vi "Experiment 11.vi"() -> ()   [LabVIEW 2026]
doc: "Experiment 11"
uses:
  <vilib>/Analysis/baseanly.llb/Mean (DBL).vi
  <vilib>/Analysis/NI_AALBase.lvlib
panel:
  out "No. Of Iterations Executed - Loop 10":i32
  out "Output - Loop 10":dbl[](array[numeric]) format="%.3f"
  out "No. Of Iterations Executed - Loop 9":i32
  out "Output - Loop 9":dbl[](array[numeric]) format="%.3f"
  out "No. Of Iterations Executed - Loop 8":i32
  out "Output - Loop 8":dbl[](array[numeric]) format="%.3f"
  out "No. Of Iterations Executed - Loop 7":i32
  out "Output - Loop 7":dbl[](array[numeric]) format="%.3f"
  out "No. Of Iterations Executed - Loop 6":i32
  out "Output - Loop 6":dbl[](array[numeric]) format="%.3f"
  out "No. Of Iterations Executed - Loop 5":i32
  out "Output - Loop 5":dbl[](array[numeric]) format="%.3f"
  out "No. Of Iterations Executed - Loop 4":i32
  out "Output - Loop 4":dbl[](array[numeric]) format="%.3f"
  out "No. Of Iterations Executed - Loop 3":i32
  out "Output - Loop 3":dbl[](array[numeric]) format="%.3f"
  out "Avg. No. Of Iterations Executed - All Loops":dbl format="%.1f"
  out "No. Of Iterations Executed - Loop 2":i32
  out "Output - Loop 2":dbl[](array[numeric]) format="%.3f"
  out "No. Of Iterations Executed - Loop 1":i32
  out "Output - Loop 1":dbl[](array[numeric]) format="%.3f"
  out "Stop VI?":bool
  # "Experiment 11"
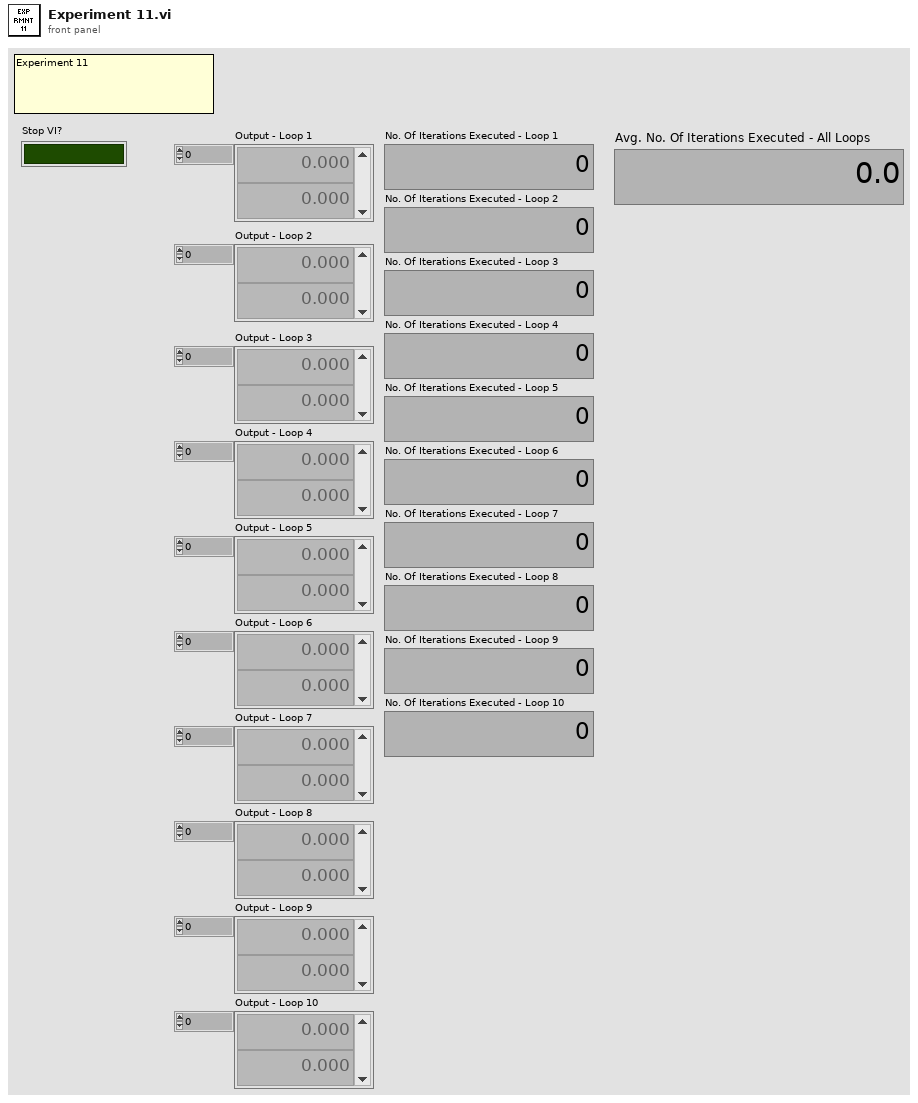
[diagram p1: front panel]
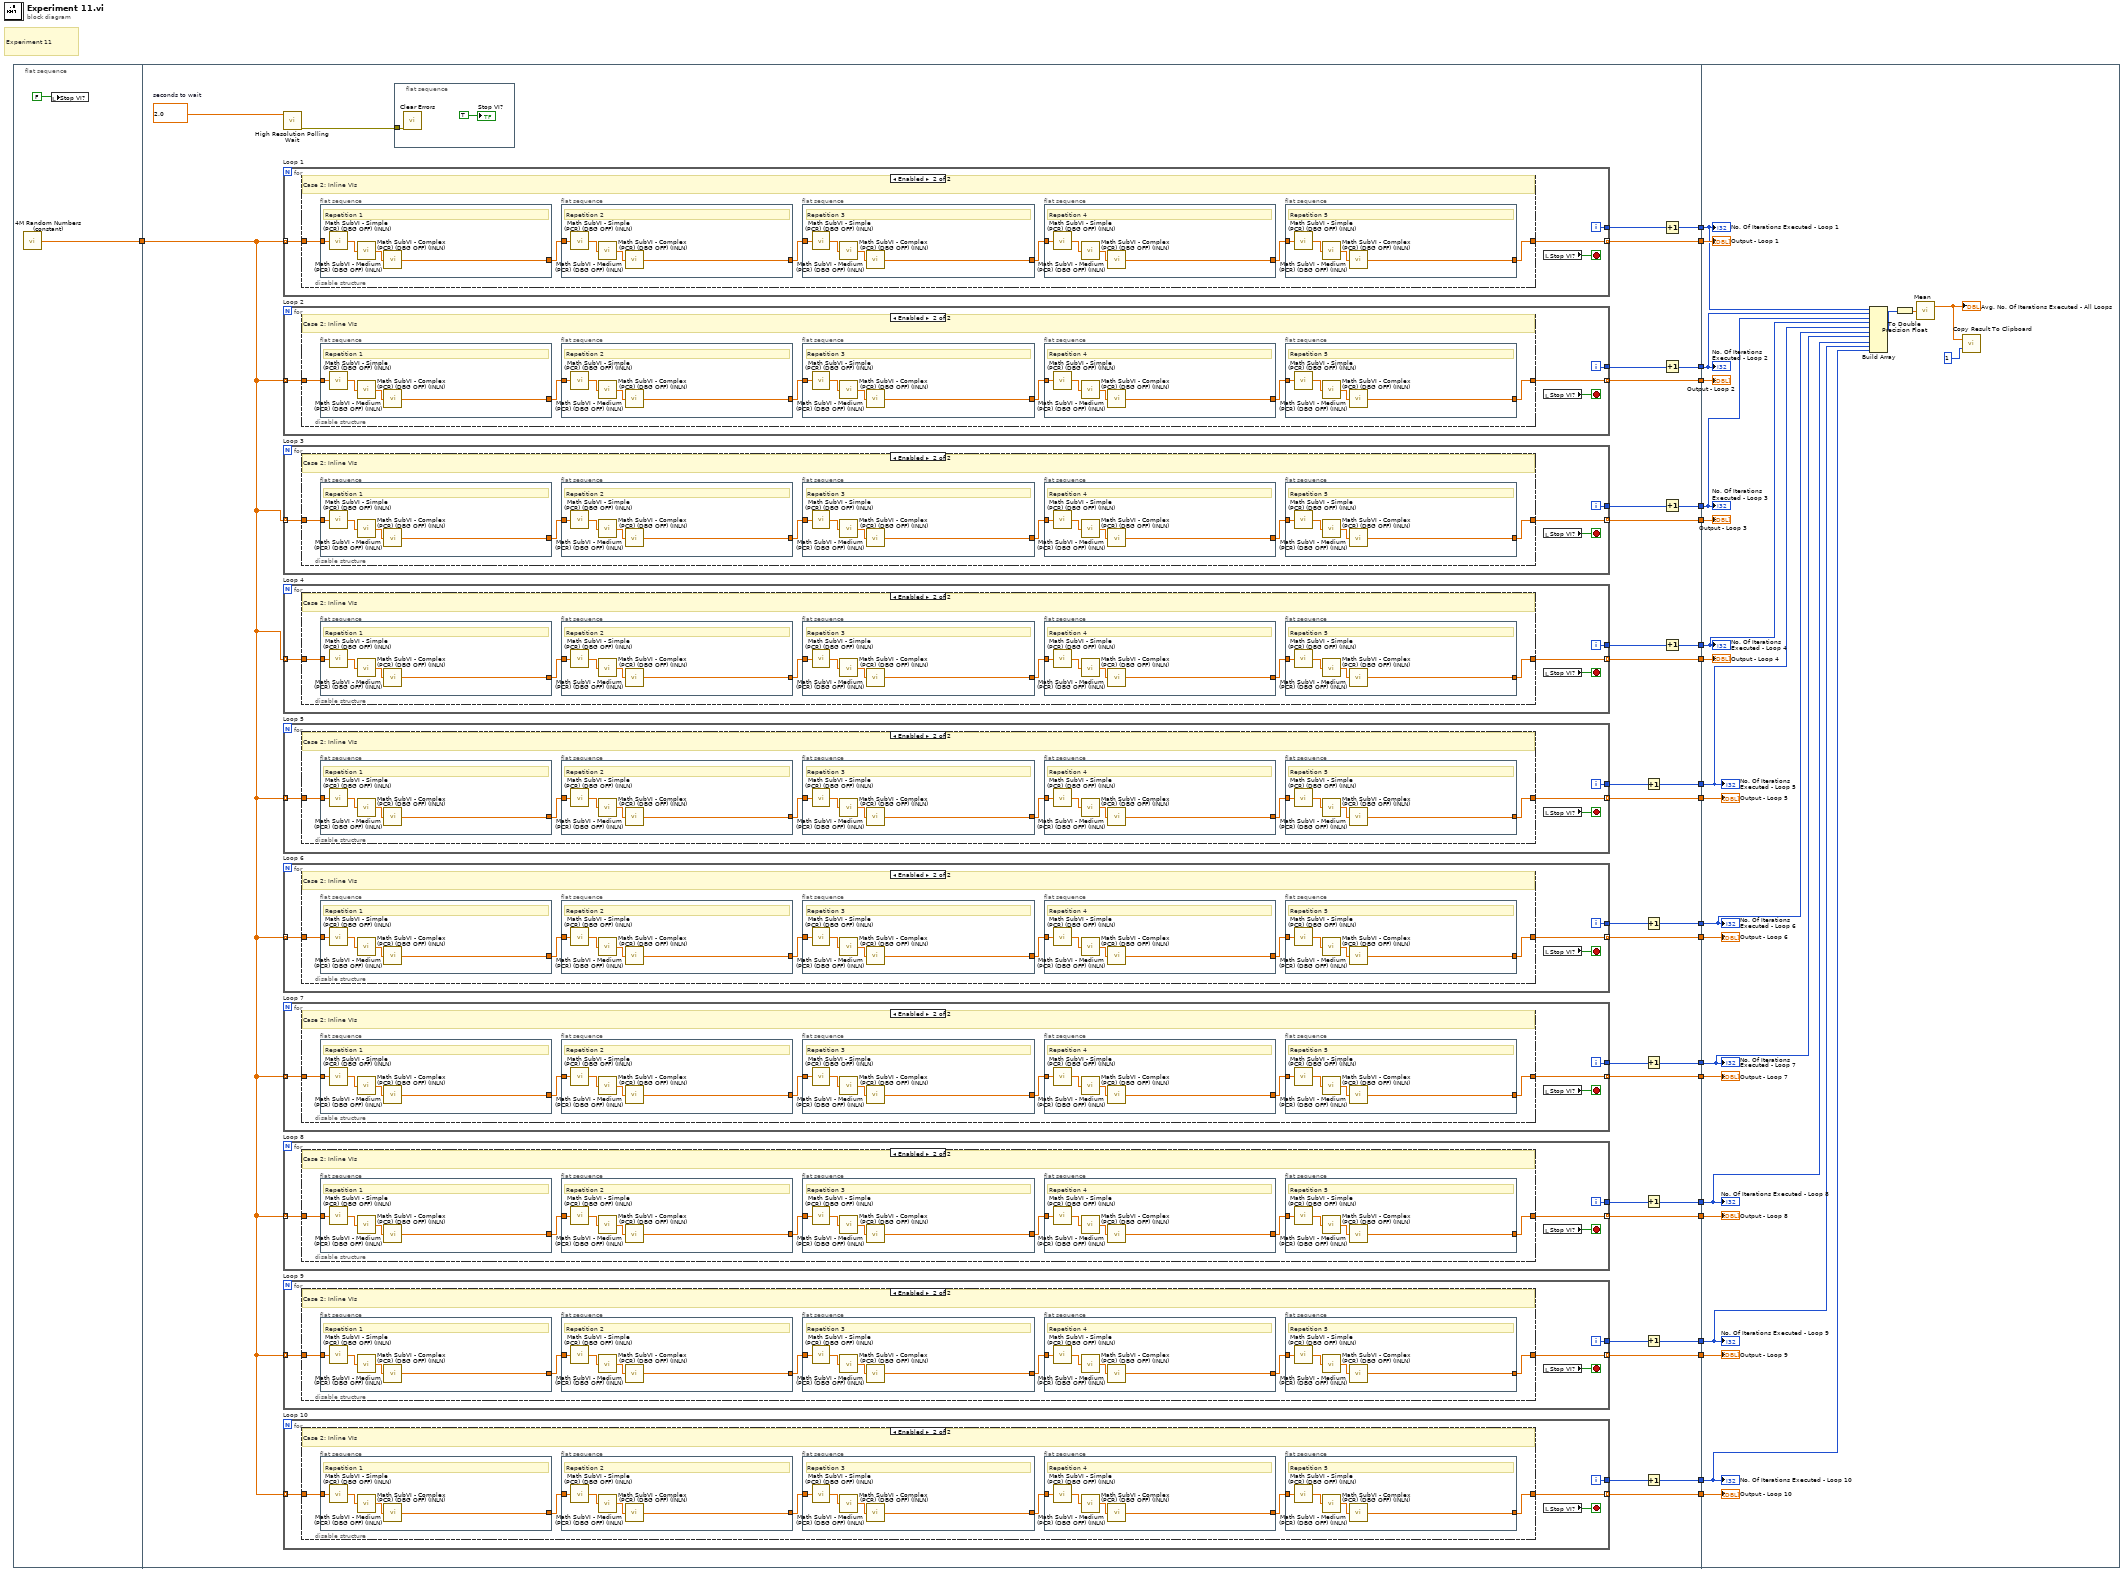
[diagram p0: block diagram]
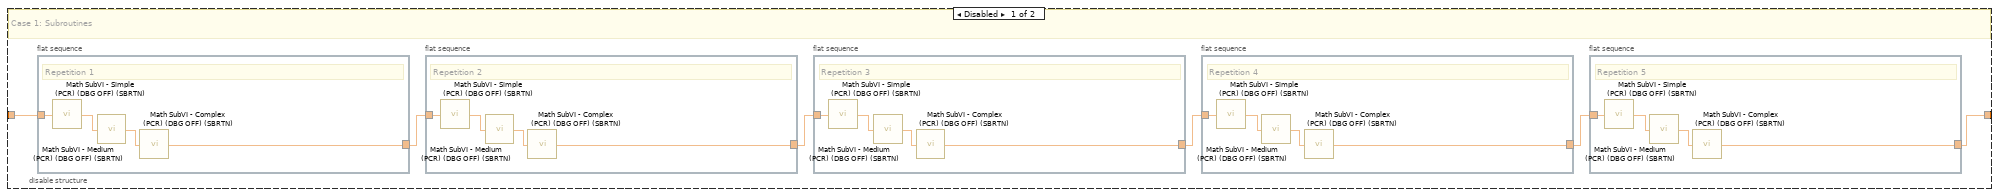
[diagram p2: hidden frame]
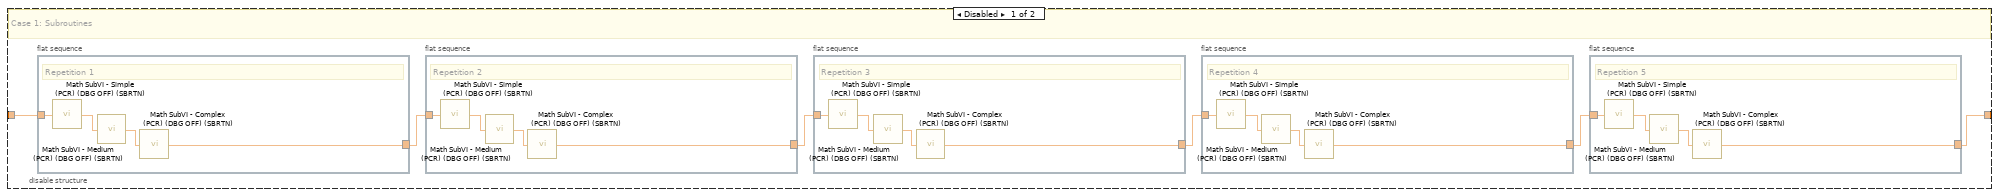
[diagram p3: hidden frame]
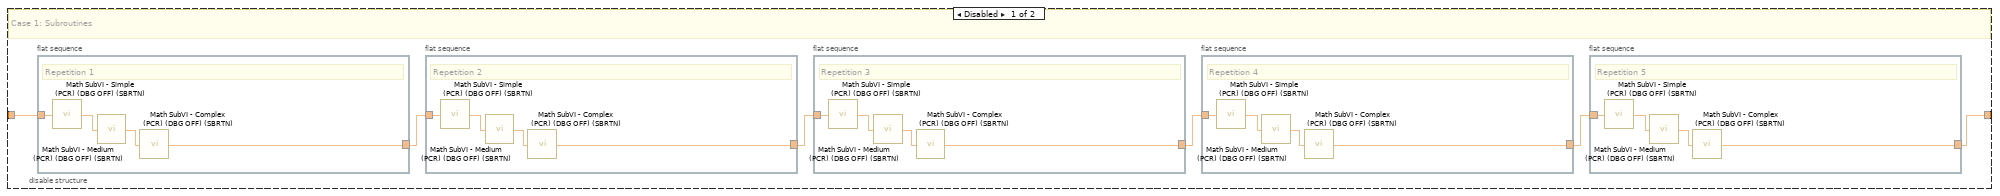
[diagram p4: hidden frame]
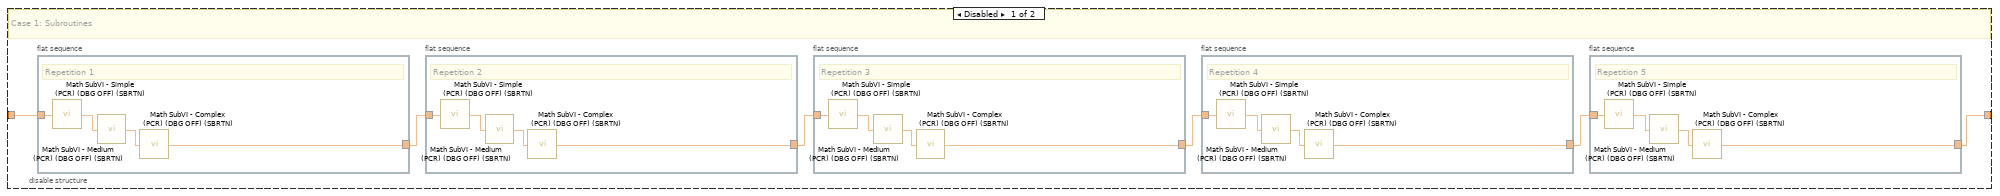
[diagram p5: hidden frame]
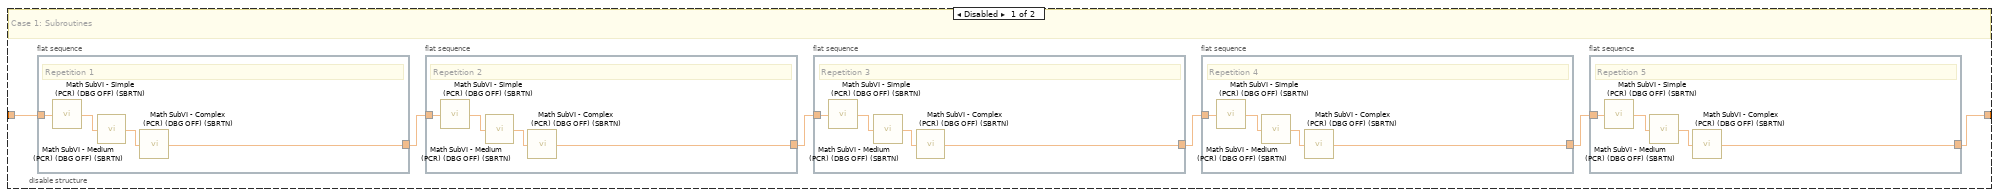
[diagram p6: hidden frame]
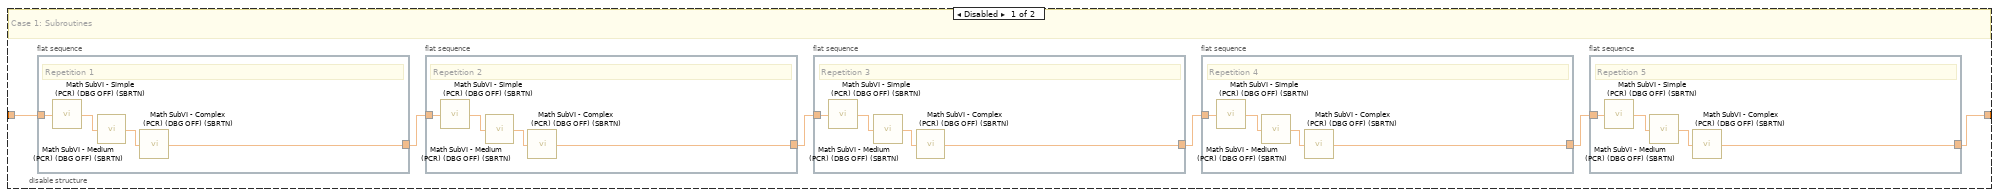
[diagram p7: hidden frame]
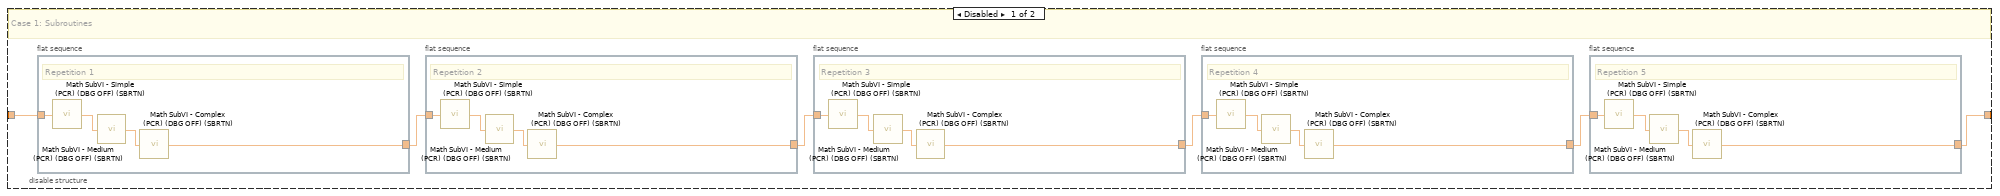
[diagram p8: hidden frame]
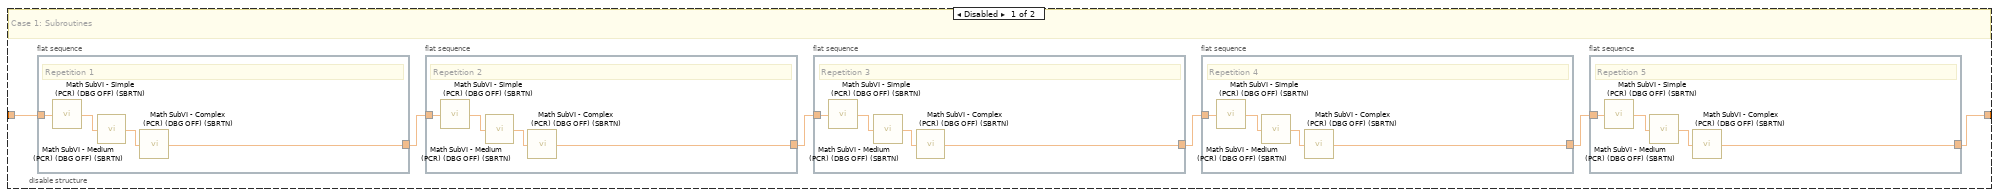
[diagram p9: hidden frame]
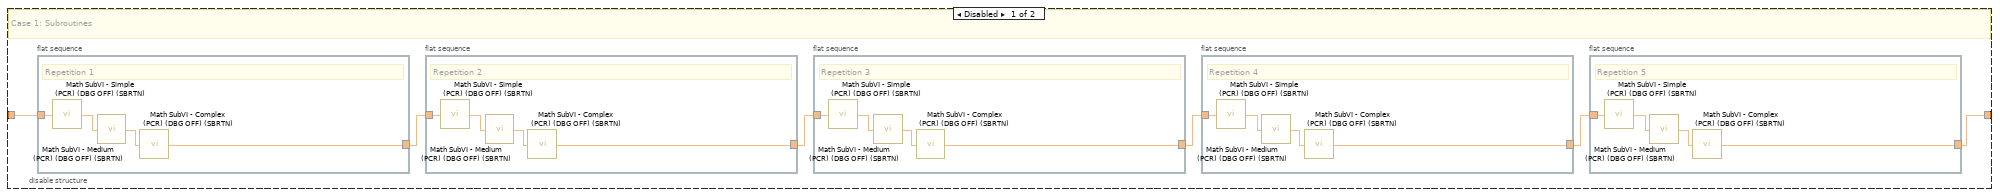
[diagram p10: hidden frame]
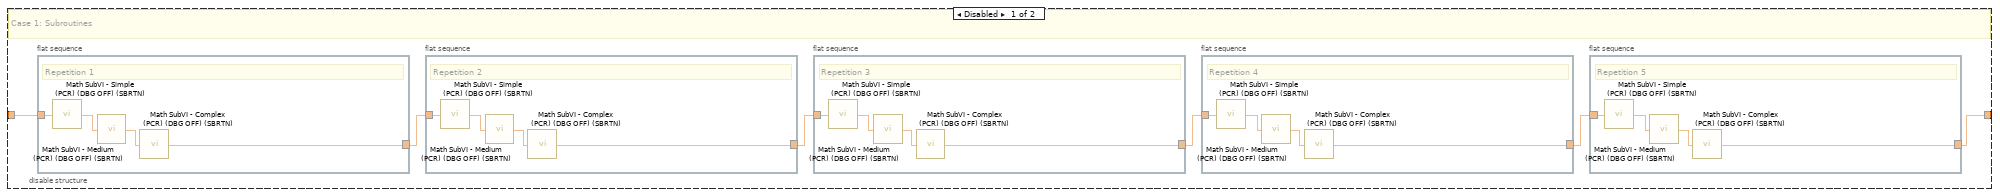
[diagram p11: hidden frame]
diagram:
  # "Experiment 11"
  n1 = flat-sequence {
    tunnel: [w22] -> w13
    tunnel: [w54] -> w21
    tunnel: [w52] -> w20
    tunnel: [w51] -> w19
    tunnel: [w46] -> w18
    tunnel: [w50] -> w17
    tunnel: [w44] -> w16
    tunnel: [w42] -> w15
    tunnel: [w49] -> w14
    tunnel: w13 -> [w48]
    tunnel: [w41] -> w12
    tunnel: [w39] -> w11
    tunnel: [w38] -> w10
    tunnel: [w24] -> w9
    tunnel: [w36] -> w8
    tunnel: [w25] -> w7
    tunnel: [w34] -> w6
    tunnel: [w26] -> w5
    tunnel: [w32] -> w4
    tunnel: [w27] -> w3
    tunnel: [w30] -> w2
    tunnel: [w28] -> w1
    tunnel: w21 -> [w642]
    tunnel: w20 -> [w640]
    tunnel: w19 -> [w639]
    tunnel: w18 -> [w641]
    tunnel: w17 -> [w634]
    tunnel: w16 -> [w637]
    tunnel: w15 -> [w636]
    tunnel: w14 -> [w633]
    tunnel: w12 -> [w630]
    tunnel: w11 -> [w624]
    tunnel: w10 -> [w629]
    tunnel: w9 -> [w623]
    tunnel: w8 -> [w628]
    tunnel: w7 -> [w622]
    tunnel: w6 -> [w627]
    tunnel: w5 -> [w621]
    tunnel: w4 -> [w626]
    tunnel: w3 -> [w620]
    tunnel: w2 -> [w625]
    tunnel: w1 -> [w619]
    frame #0 {
      n2 = call "4M Random Numbers (constant).vi"() -> ("4M Random Numbers"=w22:dbl[])
      n3 = local write "Stop VI?"(FALSE) -> ()
    }
    frame #1 {
      w56 = 2.0  # seconds to wait
      n4 = call <vilib>:"High Resolution Polling Wait.vi"("seconds to wait"=w56) -> ("error out"=w55:errorcluster)  [unwired: 10 in]
      n5 = for "Loop 1" {
        tunnel: w48 -> [w564] mode=indexing
        tunnel: [w561] -> w54 mode=indexing
        tunnel: [w562] -> w53
        i -> [w562]
        stop <- w563 stop-if-true
        n6 = disable-structure shown="Enabled" {
          disable-tunnel: w564 -> [w570 w596]
          disable-tunnel: [w569 w591] -> w561
          frame Disabled {
            # "Case 1: Subroutines"
            n7 = flat-sequence {
              tunnel: w570 -> [w590]
              tunnel: [w587] -> w565
              frame #0 {
                # "Repetition 1"
                n8 = call "Math SubVI - Simple (PCR) (DBG OFF) (SBRTN).vi"("Input"=w590) -> ("Output"=w588:dbl)
                n9 = call "Math SubVI - Medium (PCR) (DBG OFF) (SBRTN).vi"("Input"=w588) -> ("Output"=w589:dbl)
                n10 = call "Math SubVI - Complex (PCR) (DBG OFF) (SBRTN).vi"("Input"=w589) -> ("Output"=w587:dbl)
              }
            }
            n11 = flat-sequence {
              tunnel: w565 -> [w586]
              tunnel: [w583] -> w568
              frame #0 {
                # "Repetition 2"
                n12 = call "Math SubVI - Simple (PCR) (DBG OFF) (SBRTN).vi"("Input"=w586) -> ("Output"=w584:dbl)
                n13 = call "Math SubVI - Medium (PCR) (DBG OFF) (SBRTN).vi"("Input"=w584) -> ("Output"=w585:dbl)
                n14 = call "Math SubVI - Complex (PCR) (DBG OFF) (SBRTN).vi"("Input"=w585) -> ("Output"=w583:dbl)
              }
            }
            n15 = flat-sequence {
              tunnel: w568 -> [w582]
              tunnel: [w579] -> w567
              frame #0 {
                # "Repetition 3"
                n16 = call "Math SubVI - Simple (PCR) (DBG OFF) (SBRTN).vi"("Input"=w582) -> ("Output"=w580:dbl)
                n17 = call "Math SubVI - Medium (PCR) (DBG OFF) (SBRTN).vi"("Input"=w580) -> ("Output"=w581:dbl)
                n18 = call "Math SubVI - Complex (PCR) (DBG OFF) (SBRTN).vi"("Input"=w581) -> ("Output"=w579:dbl)
              }
            }
            n19 = flat-sequence {
              tunnel: w567 -> [w578]
              tunnel: [w575] -> w566
              frame #0 {
                # "Repetition 4"
                n20 = call "Math SubVI - Simple (PCR) (DBG OFF) (SBRTN).vi"("Input"=w578) -> ("Output"=w576:dbl)
                n21 = call "Math SubVI - Medium (PCR) (DBG OFF) (SBRTN).vi"("Input"=w576) -> ("Output"=w577:dbl)
                n22 = call "Math SubVI - Complex (PCR) (DBG OFF) (SBRTN).vi"("Input"=w577) -> ("Output"=w575:dbl)
              }
            }
            n23 = flat-sequence {
              tunnel: w566 -> [w574]
              tunnel: [w571] -> w569
              frame #0 {
                # "Repetition 5"
                n24 = call "Math SubVI - Simple (PCR) (DBG OFF) (SBRTN).vi"("Input"=w574) -> ("Output"=w572:dbl)
                n25 = call "Math SubVI - Medium (PCR) (DBG OFF) (SBRTN).vi"("Input"=w572) -> ("Output"=w573:dbl)
                n26 = call "Math SubVI - Complex (PCR) (DBG OFF) (SBRTN).vi"("Input"=w573) -> ("Output"=w571:dbl)
              }
            }
          }
          frame Enabled {
            # "Case 2: Inline VIs"
            n27 = flat-sequence {
              tunnel: w596 -> [w616]
              tunnel: [w613] -> w595
              frame #0 {
                # "Repetition 1"
                n28 = call "Math SubVI - Simple (PCR) (DBG OFF) (INLN).vi"("Input"=w616) -> ("Output"=w614:dbl)
                n29 = call "Math SubVI - Medium (PCR) (DBG OFF) (INLN).vi"("Input"=w614) -> ("Output"=w615:dbl)
                n30 = call "Math SubVI - Complex (PCR) (DBG OFF) (INLN).vi"("Input"=w615) -> ("Output"=w613:dbl)
              }
            }
            n31 = flat-sequence {
              tunnel: w595 -> [w612]
              tunnel: [w609] -> w594
              frame #0 {
                # "Repetition 2"
                n32 = call "Math SubVI - Simple (PCR) (DBG OFF) (INLN).vi"("Input"=w612) -> ("Output"=w610:dbl)
                n33 = call "Math SubVI - Medium (PCR) (DBG OFF) (INLN).vi"("Input"=w610) -> ("Output"=w611:dbl)
                n34 = call "Math SubVI - Complex (PCR) (DBG OFF) (INLN).vi"("Input"=w611) -> ("Output"=w609:dbl)
              }
            }
            n35 = flat-sequence {
              tunnel: w594 -> [w608]
              tunnel: [w605] -> w593
              frame #0 {
                # "Repetition 3"
                n36 = call "Math SubVI - Simple (PCR) (DBG OFF) (INLN).vi"("Input"=w608) -> ("Output"=w606:dbl)
                n37 = call "Math SubVI - Medium (PCR) (DBG OFF) (INLN).vi"("Input"=w606) -> ("Output"=w607:dbl)
                n38 = call "Math SubVI - Complex (PCR) (DBG OFF) (INLN).vi"("Input"=w607) -> ("Output"=w605:dbl)
              }
            }
            n39 = flat-sequence {
              tunnel: w593 -> [w604]
              tunnel: [w601] -> w592
              frame #0 {
                # "Repetition 4"
                n40 = call "Math SubVI - Simple (PCR) (DBG OFF) (INLN).vi"("Input"=w604) -> ("Output"=w602:dbl)
                n41 = call "Math SubVI - Medium (PCR) (DBG OFF) (INLN).vi"("Input"=w602) -> ("Output"=w603:dbl)
                n42 = call "Math SubVI - Complex (PCR) (DBG OFF) (INLN).vi"("Input"=w603) -> ("Output"=w601:dbl)
              }
            }
            n43 = flat-sequence {
              tunnel: w592 -> [w600]
              tunnel: [w597] -> w591
              frame #0 {
                # "Repetition 5"
                n44 = call "Math SubVI - Simple (PCR) (DBG OFF) (INLN).vi"("Input"=w600) -> ("Output"=w598:dbl)
                n45 = call "Math SubVI - Medium (PCR) (DBG OFF) (INLN).vi"("Input"=w598) -> ("Output"=w599:dbl)
                n46 = call "Math SubVI - Complex (PCR) (DBG OFF) (INLN).vi"("Input"=w599) -> ("Output"=w597:dbl)
              }
            }
          }
        }
        n47 = local read "Stop VI?"() -> (w563:bool)
      }
      n48 = for "Loop 2" {
        tunnel: w48 -> [w508] mode=indexing
        tunnel: [w505] -> w46 mode=indexing
        tunnel: [w506] -> w47
        i -> [w506]
        stop <- w507 stop-if-true
        n49 = disable-structure shown="Enabled" {
          disable-tunnel: w508 -> [w514 w540]
          disable-tunnel: [w513 w535] -> w505
          frame Disabled {
            # "Case 1: Subroutines"
            n50 = flat-sequence {
              tunnel: w514 -> [w534]
              tunnel: [w531] -> w509
              frame #0 {
                # "Repetition 1"
                n51 = call "Math SubVI - Simple (PCR) (DBG OFF) (SBRTN).vi"("Input"=w534) -> ("Output"=w532:dbl)
                n52 = call "Math SubVI - Medium (PCR) (DBG OFF) (SBRTN).vi"("Input"=w532) -> ("Output"=w533:dbl)
                n53 = call "Math SubVI - Complex (PCR) (DBG OFF) (SBRTN).vi"("Input"=w533) -> ("Output"=w531:dbl)
              }
            }
            n54 = flat-sequence {
              tunnel: w509 -> [w530]
              tunnel: [w527] -> w512
              frame #0 {
                # "Repetition 2"
                n55 = call "Math SubVI - Simple (PCR) (DBG OFF) (SBRTN).vi"("Input"=w530) -> ("Output"=w528:dbl)
                n56 = call "Math SubVI - Medium (PCR) (DBG OFF) (SBRTN).vi"("Input"=w528) -> ("Output"=w529:dbl)
                n57 = call "Math SubVI - Complex (PCR) (DBG OFF) (SBRTN).vi"("Input"=w529) -> ("Output"=w527:dbl)
              }
            }
            n58 = flat-sequence {
              tunnel: w512 -> [w526]
              tunnel: [w523] -> w511
              frame #0 {
                # "Repetition 3"
                n59 = call "Math SubVI - Simple (PCR) (DBG OFF) (SBRTN).vi"("Input"=w526) -> ("Output"=w524:dbl)
                n60 = call "Math SubVI - Medium (PCR) (DBG OFF) (SBRTN).vi"("Input"=w524) -> ("Output"=w525:dbl)
                n61 = call "Math SubVI - Complex (PCR) (DBG OFF) (SBRTN).vi"("Input"=w525) -> ("Output"=w523:dbl)
              }
            }
            n62 = flat-sequence {
              tunnel: w511 -> [w522]
              tunnel: [w519] -> w510
              frame #0 {
                # "Repetition 4"
                n63 = call "Math SubVI - Simple (PCR) (DBG OFF) (SBRTN).vi"("Input"=w522) -> ("Output"=w520:dbl)
                n64 = call "Math SubVI - Medium (PCR) (DBG OFF) (SBRTN).vi"("Input"=w520) -> ("Output"=w521:dbl)
                n65 = call "Math SubVI - Complex (PCR) (DBG OFF) (SBRTN).vi"("Input"=w521) -> ("Output"=w519:dbl)
              }
            }
            n66 = flat-sequence {
              tunnel: w510 -> [w518]
              tunnel: [w515] -> w513
              frame #0 {
                # "Repetition 5"
                n67 = call "Math SubVI - Simple (PCR) (DBG OFF) (SBRTN).vi"("Input"=w518) -> ("Output"=w516:dbl)
                n68 = call "Math SubVI - Medium (PCR) (DBG OFF) (SBRTN).vi"("Input"=w516) -> ("Output"=w517:dbl)
                n69 = call "Math SubVI - Complex (PCR) (DBG OFF) (SBRTN).vi"("Input"=w517) -> ("Output"=w515:dbl)
              }
            }
          }
          frame Enabled {
            # "Case 2: Inline VIs"
            n70 = flat-sequence {
              tunnel: w540 -> [w560]
              tunnel: [w557] -> w539
              frame #0 {
                # "Repetition 1"
                n71 = call "Math SubVI - Simple (PCR) (DBG OFF) (INLN).vi"("Input"=w560) -> ("Output"=w558:dbl)
                n72 = call "Math SubVI - Medium (PCR) (DBG OFF) (INLN).vi"("Input"=w558) -> ("Output"=w559:dbl)
                n73 = call "Math SubVI - Complex (PCR) (DBG OFF) (INLN).vi"("Input"=w559) -> ("Output"=w557:dbl)
              }
            }
            n74 = flat-sequence {
              tunnel: w539 -> [w556]
              tunnel: [w553] -> w538
              frame #0 {
                # "Repetition 2"
                n75 = call "Math SubVI - Simple (PCR) (DBG OFF) (INLN).vi"("Input"=w556) -> ("Output"=w554:dbl)
                n76 = call "Math SubVI - Medium (PCR) (DBG OFF) (INLN).vi"("Input"=w554) -> ("Output"=w555:dbl)
                n77 = call "Math SubVI - Complex (PCR) (DBG OFF) (INLN).vi"("Input"=w555) -> ("Output"=w553:dbl)
              }
            }
            n78 = flat-sequence {
              tunnel: w538 -> [w552]
              tunnel: [w549] -> w537
              frame #0 {
                # "Repetition 3"
                n79 = call "Math SubVI - Simple (PCR) (DBG OFF) (INLN).vi"("Input"=w552) -> ("Output"=w550:dbl)
                n80 = call "Math SubVI - Medium (PCR) (DBG OFF) (INLN).vi"("Input"=w550) -> ("Output"=w551:dbl)
                n81 = call "Math SubVI - Complex (PCR) (DBG OFF) (INLN).vi"("Input"=w551) -> ("Output"=w549:dbl)
              }
            }
            n82 = flat-sequence {
              tunnel: w537 -> [w548]
              tunnel: [w545] -> w536
              frame #0 {
                # "Repetition 4"
                n83 = call "Math SubVI - Simple (PCR) (DBG OFF) (INLN).vi"("Input"=w548) -> ("Output"=w546:dbl)
                n84 = call "Math SubVI - Medium (PCR) (DBG OFF) (INLN).vi"("Input"=w546) -> ("Output"=w547:dbl)
                n85 = call "Math SubVI - Complex (PCR) (DBG OFF) (INLN).vi"("Input"=w547) -> ("Output"=w545:dbl)
              }
            }
            n86 = flat-sequence {
              tunnel: w536 -> [w544]
              tunnel: [w541] -> w535
              frame #0 {
                # "Repetition 5"
                n87 = call "Math SubVI - Simple (PCR) (DBG OFF) (INLN).vi"("Input"=w544) -> ("Output"=w542:dbl)
                n88 = call "Math SubVI - Medium (PCR) (DBG OFF) (INLN).vi"("Input"=w542) -> ("Output"=w543:dbl)
                n89 = call "Math SubVI - Complex (PCR) (DBG OFF) (INLN).vi"("Input"=w543) -> ("Output"=w541:dbl)
              }
            }
          }
        }
        n90 = local read "Stop VI?"() -> (w507:bool)
      }
      n91 = for "Loop 3" {
        tunnel: w48 -> [w452] mode=indexing
        tunnel: [w449] -> w44 mode=indexing
        tunnel: [w450] -> w45
        i -> [w450]
        stop <- w451 stop-if-true
        n92 = disable-structure shown="Enabled" {
          disable-tunnel: w452 -> [w458 w484]
          disable-tunnel: [w457 w479] -> w449
          frame Disabled {
            # "Case 1: Subroutines"
            n93 = flat-sequence {
              tunnel: w458 -> [w478]
              tunnel: [w475] -> w453
              frame #0 {
                # "Repetition 1"
                n94 = call "Math SubVI - Simple (PCR) (DBG OFF) (SBRTN).vi"("Input"=w478) -> ("Output"=w476:dbl)
                n95 = call "Math SubVI - Medium (PCR) (DBG OFF) (SBRTN).vi"("Input"=w476) -> ("Output"=w477:dbl)
                n96 = call "Math SubVI - Complex (PCR) (DBG OFF) (SBRTN).vi"("Input"=w477) -> ("Output"=w475:dbl)
              }
            }
            n97 = flat-sequence {
              tunnel: w453 -> [w474]
              tunnel: [w471] -> w456
              frame #0 {
                # "Repetition 2"
                n98 = call "Math SubVI - Simple (PCR) (DBG OFF) (SBRTN).vi"("Input"=w474) -> ("Output"=w472:dbl)
                n99 = call "Math SubVI - Medium (PCR) (DBG OFF) (SBRTN).vi"("Input"=w472) -> ("Output"=w473:dbl)
                n100 = call "Math SubVI - Complex (PCR) (DBG OFF) (SBRTN).vi"("Input"=w473) -> ("Output"=w471:dbl)
              }
            }
            n101 = flat-sequence {
              tunnel: w456 -> [w470]
              tunnel: [w467] -> w455
              frame #0 {
                # "Repetition 3"
                n102 = call "Math SubVI - Simple (PCR) (DBG OFF) (SBRTN).vi"("Input"=w470) -> ("Output"=w468:dbl)
                n103 = call "Math SubVI - Medium (PCR) (DBG OFF) (SBRTN).vi"("Input"=w468) -> ("Output"=w469:dbl)
                n104 = call "Math SubVI - Complex (PCR) (DBG OFF) (SBRTN).vi"("Input"=w469) -> ("Output"=w467:dbl)
              }
            }
            n105 = flat-sequence {
              tunnel: w455 -> [w466]
              tunnel: [w463] -> w454
              frame #0 {
                # "Repetition 4"
                n106 = call "Math SubVI - Simple (PCR) (DBG OFF) (SBRTN).vi"("Input"=w466) -> ("Output"=w464:dbl)
                n107 = call "Math SubVI - Medium (PCR) (DBG OFF) (SBRTN).vi"("Input"=w464) -> ("Output"=w465:dbl)
                n108 = call "Math SubVI - Complex (PCR) (DBG OFF) (SBRTN).vi"("Input"=w465) -> ("Output"=w463:dbl)
              }
            }
            n109 = flat-sequence {
              tunnel: w454 -> [w462]
              tunnel: [w459] -> w457
              frame #0 {
                # "Repetition 5"
                n110 = call "Math SubVI - Simple (PCR) (DBG OFF) (SBRTN).vi"("Input"=w462) -> ("Output"=w460:dbl)
                n111 = call "Math SubVI - Medium (PCR) (DBG OFF) (SBRTN).vi"("Input"=w460) -> ("Output"=w461:dbl)
                n112 = call "Math SubVI - Complex (PCR) (DBG OFF) (SBRTN).vi"("Input"=w461) -> ("Output"=w459:dbl)
              }
            }
          }
          frame Enabled {
            # "Case 2: Inline VIs"
            n113 = flat-sequence {
              tunnel: w484 -> [w504]
              tunnel: [w501] -> w483
              frame #0 {
                # "Repetition 1"
                n114 = call "Math SubVI - Simple (PCR) (DBG OFF) (INLN).vi"("Input"=w504) -> ("Output"=w502:dbl)
                n115 = call "Math SubVI - Medium (PCR) (DBG OFF) (INLN).vi"("Input"=w502) -> ("Output"=w503:dbl)
                n116 = call "Math SubVI - Complex (PCR) (DBG OFF) (INLN).vi"("Input"=w503) -> ("Output"=w501:dbl)
              }
            }
            n117 = flat-sequence {
              tunnel: w483 -> [w500]
              tunnel: [w497] -> w482
              frame #0 {
                # "Repetition 2"
                n118 = call "Math SubVI - Simple (PCR) (DBG OFF) (INLN).vi"("Input"=w500) -> ("Output"=w498:dbl)
                n119 = call "Math SubVI - Medium (PCR) (DBG OFF) (INLN).vi"("Input"=w498) -> ("Output"=w499:dbl)
                n120 = call "Math SubVI - Complex (PCR) (DBG OFF) (INLN).vi"("Input"=w499) -> ("Output"=w497:dbl)
              }
            }
            n121 = flat-sequence {
              tunnel: w482 -> [w496]
              tunnel: [w493] -> w481
              frame #0 {
                # "Repetition 3"
                n122 = call "Math SubVI - Simple (PCR) (DBG OFF) (INLN).vi"("Input"=w496) -> ("Output"=w494:dbl)
                n123 = call "Math SubVI - Medium (PCR) (DBG OFF) (INLN).vi"("Input"=w494) -> ("Output"=w495:dbl)
                n124 = call "Math SubVI - Complex (PCR) (DBG OFF) (INLN).vi"("Input"=w495) -> ("Output"=w493:dbl)
              }
            }
            n125 = flat-sequence {
              tunnel: w481 -> [w492]
              tunnel: [w489] -> w480
              frame #0 {
                # "Repetition 4"
                n126 = call "Math SubVI - Simple (PCR) (DBG OFF) (INLN).vi"("Input"=w492) -> ("Output"=w490:dbl)
                n127 = call "Math SubVI - Medium (PCR) (DBG OFF) (INLN).vi"("Input"=w490) -> ("Output"=w491:dbl)
                n128 = call "Math SubVI - Complex (PCR) (DBG OFF) (INLN).vi"("Input"=w491) -> ("Output"=w489:dbl)
              }
            }
            n129 = flat-sequence {
              tunnel: w480 -> [w488]
              tunnel: [w485] -> w479
              frame #0 {
                # "Repetition 5"
                n130 = call "Math SubVI - Simple (PCR) (DBG OFF) (INLN).vi"("Input"=w488) -> ("Output"=w486:dbl)
                n131 = call "Math SubVI - Medium (PCR) (DBG OFF) (INLN).vi"("Input"=w486) -> ("Output"=w487:dbl)
                n132 = call "Math SubVI - Complex (PCR) (DBG OFF) (INLN).vi"("Input"=w487) -> ("Output"=w485:dbl)
              }
            }
          }
        }
        n133 = local read "Stop VI?"() -> (w451:bool)
      }
      n134 = for "Loop 4" {
        tunnel: w48 -> [w396] mode=indexing
        tunnel: [w393] -> w42 mode=indexing
        tunnel: [w394] -> w43
        i -> [w394]
        stop <- w395 stop-if-true
        n135 = disable-structure shown="Enabled" {
          disable-tunnel: w396 -> [w402 w428]
          disable-tunnel: [w401 w423] -> w393
          frame Disabled {
            # "Case 1: Subroutines"
            n136 = flat-sequence {
              tunnel: w402 -> [w422]
              tunnel: [w419] -> w397
              frame #0 {
                # "Repetition 1"
                n137 = call "Math SubVI - Simple (PCR) (DBG OFF) (SBRTN).vi"("Input"=w422) -> ("Output"=w420:dbl)
                n138 = call "Math SubVI - Medium (PCR) (DBG OFF) (SBRTN).vi"("Input"=w420) -> ("Output"=w421:dbl)
                n139 = call "Math SubVI - Complex (PCR) (DBG OFF) (SBRTN).vi"("Input"=w421) -> ("Output"=w419:dbl)
              }
            }
            n140 = flat-sequence {
              tunnel: w397 -> [w418]
              tunnel: [w415] -> w400
              frame #0 {
                # "Repetition 2"
                n141 = call "Math SubVI - Simple (PCR) (DBG OFF) (SBRTN).vi"("Input"=w418) -> ("Output"=w416:dbl)
                n142 = call "Math SubVI - Medium (PCR) (DBG OFF) (SBRTN).vi"("Input"=w416) -> ("Output"=w417:dbl)
                n143 = call "Math SubVI - Complex (PCR) (DBG OFF) (SBRTN).vi"("Input"=w417) -> ("Output"=w415:dbl)
              }
            }
            n144 = flat-sequence {
              tunnel: w400 -> [w414]
              tunnel: [w411] -> w399
              frame #0 {
                # "Repetition 3"
                n145 = call "Math SubVI - Simple (PCR) (DBG OFF) (SBRTN).vi"("Input"=w414) -> ("Output"=w412:dbl)
                n146 = call "Math SubVI - Medium (PCR) (DBG OFF) (SBRTN).vi"("Input"=w412) -> ("Output"=w413:dbl)
                n147 = call "Math SubVI - Complex (PCR) (DBG OFF) (SBRTN).vi"("Input"=w413) -> ("Output"=w411:dbl)
              }
            }
            n148 = flat-sequence {
              tunnel: w399 -> [w410]
              tunnel: [w407] -> w398
              frame #0 {
                # "Repetition 4"
                n149 = call "Math SubVI - Simple (PCR) (DBG OFF) (SBRTN).vi"("Input"=w410) -> ("Output"=w408:dbl)
                n150 = call "Math SubVI - Medium (PCR) (DBG OFF) (SBRTN).vi"("Input"=w408) -> ("Output"=w409:dbl)
                n151 = call "Math SubVI - Complex (PCR) (DBG OFF) (SBRTN).vi"("Input"=w409) -> ("Output"=w407:dbl)
              }
            }
            n152 = flat-sequence {
              tunnel: w398 -> [w406]
              tunnel: [w403] -> w401
              frame #0 {
                # "Repetition 5"
                n153 = call "Math SubVI - Simple (PCR) (DBG OFF) (SBRTN).vi"("Input"=w406) -> ("Output"=w404:dbl)
                n154 = call "Math SubVI - Medium (PCR) (DBG OFF) (SBRTN).vi"("Input"=w404) -> ("Output"=w405:dbl)
                n155 = call "Math SubVI - Complex (PCR) (DBG OFF) (SBRTN).vi"("Input"=w405) -> ("Output"=w403:dbl)
              }
            }
          }
          frame Enabled {
            # "Case 2: Inline VIs"
            n156 = flat-sequence {
              tunnel: w428 -> [w448]
              tunnel: [w445] -> w427
              frame #0 {
                # "Repetition 1"
                n157 = call "Math SubVI - Simple (PCR) (DBG OFF) (INLN).vi"("Input"=w448) -> ("Output"=w446:dbl)
                n158 = call "Math SubVI - Medium (PCR) (DBG OFF) (INLN).vi"("Input"=w446) -> ("Output"=w447:dbl)
                n159 = call "Math SubVI - Complex (PCR) (DBG OFF) (INLN).vi"("Input"=w447) -> ("Output"=w445:dbl)
              }
            }
            n160 = flat-sequence {
              tunnel: w427 -> [w444]
              tunnel: [w441] -> w426
              frame #0 {
                # "Repetition 2"
                n161 = call "Math SubVI - Simple (PCR) (DBG OFF) (INLN).vi"("Input"=w444) -> ("Output"=w442:dbl)
                n162 = call "Math SubVI - Medium (PCR) (DBG OFF) (INLN).vi"("Input"=w442) -> ("Output"=w443:dbl)
                n163 = call "Math SubVI - Complex (PCR) (DBG OFF) (INLN).vi"("Input"=w443) -> ("Output"=w441:dbl)
              }
            }
            n164 = flat-sequence {
              tunnel: w426 -> [w440]
              tunnel: [w437] -> w425
              frame #0 {
                # "Repetition 3"
                n165 = call "Math SubVI - Simple (PCR) (DBG OFF) (INLN).vi"("Input"=w440) -> ("Output"=w438:dbl)
                n166 = call "Math SubVI - Medium (PCR) (DBG OFF) (INLN).vi"("Input"=w438) -> ("Output"=w439:dbl)
                n167 = call "Math SubVI - Complex (PCR) (DBG OFF) (INLN).vi"("Input"=w439) -> ("Output"=w437:dbl)
              }
            }
            n168 = flat-sequence {
              tunnel: w425 -> [w436]
              tunnel: [w433] -> w424
              frame #0 {
                # "Repetition 4"
                n169 = call "Math SubVI - Simple (PCR) (DBG OFF) (INLN).vi"("Input"=w436) -> ("Output"=w434:dbl)
                n170 = call "Math SubVI - Medium (PCR) (DBG OFF) (INLN).vi"("Input"=w434) -> ("Output"=w435:dbl)
                n171 = call "Math SubVI - Complex (PCR) (DBG OFF) (INLN).vi"("Input"=w435) -> ("Output"=w433:dbl)
              }
            }
            n172 = flat-sequence {
              tunnel: w424 -> [w432]
              tunnel: [w429] -> w423
              frame #0 {
                # "Repetition 5"
                n173 = call "Math SubVI - Simple (PCR) (DBG OFF) (INLN).vi"("Input"=w432) -> ("Output"=w430:dbl)
                n174 = call "Math SubVI - Medium (PCR) (DBG OFF) (INLN).vi"("Input"=w430) -> ("Output"=w431:dbl)
                n175 = call "Math SubVI - Complex (PCR) (DBG OFF) (INLN).vi"("Input"=w431) -> ("Output"=w429:dbl)
              }
            }
          }
        }
        n176 = local read "Stop VI?"() -> (w395:bool)
      }
      n177 = for "Loop 5" {
        tunnel: w48 -> [w340] mode=indexing
        tunnel: [w337] -> w41 mode=indexing
        tunnel: [w338] -> w40
        i -> [w338]
        stop <- w339 stop-if-true
        n178 = disable-structure shown="Enabled" {
          disable-tunnel: w340 -> [w346 w372]
          disable-tunnel: [w345 w367] -> w337
          frame Disabled {
            # "Case 1: Subroutines"
            n179 = flat-sequence {
              tunnel: w346 -> [w366]
              tunnel: [w363] -> w341
              frame #0 {
                # "Repetition 1"
                n180 = call "Math SubVI - Simple (PCR) (DBG OFF) (SBRTN).vi"("Input"=w366) -> ("Output"=w364:dbl)
                n181 = call "Math SubVI - Medium (PCR) (DBG OFF) (SBRTN).vi"("Input"=w364) -> ("Output"=w365:dbl)
                n182 = call "Math SubVI - Complex (PCR) (DBG OFF) (SBRTN).vi"("Input"=w365) -> ("Output"=w363:dbl)
              }
            }
            n183 = flat-sequence {
              tunnel: w341 -> [w362]
              tunnel: [w359] -> w344
              frame #0 {
                # "Repetition 2"
                n184 = call "Math SubVI - Simple (PCR) (DBG OFF) (SBRTN).vi"("Input"=w362) -> ("Output"=w360:dbl)
                n185 = call "Math SubVI - Medium (PCR) (DBG OFF) (SBRTN).vi"("Input"=w360) -> ("Output"=w361:dbl)
                n186 = call "Math SubVI - Complex (PCR) (DBG OFF) (SBRTN).vi"("Input"=w361) -> ("Output"=w359:dbl)
              }
            }
            n187 = flat-sequence {
              tunnel: w344 -> [w358]
              tunnel: [w355] -> w343
              frame #0 {
                # "Repetition 3"
                n188 = call "Math SubVI - Simple (PCR) (DBG OFF) (SBRTN).vi"("Input"=w358) -> ("Output"=w356:dbl)
                n189 = call "Math SubVI - Medium (PCR) (DBG OFF) (SBRTN).vi"("Input"=w356) -> ("Output"=w357:dbl)
                n190 = call "Math SubVI - Complex (PCR) (DBG OFF) (SBRTN).vi"("Input"=w357) -> ("Output"=w355:dbl)
              }
            }
            n191 = flat-sequence {
              tunnel: w343 -> [w354]
              tunnel: [w351] -> w342
              frame #0 {
                # "Repetition 4"
                n192 = call "Math SubVI - Simple (PCR) (DBG OFF) (SBRTN).vi"("Input"=w354) -> ("Output"=w352:dbl)
                n193 = call "Math SubVI - Medium (PCR) (DBG OFF) (SBRTN).vi"("Input"=w352) -> ("Output"=w353:dbl)
                n194 = call "Math SubVI - Complex (PCR) (DBG OFF) (SBRTN).vi"("Input"=w353) -> ("Output"=w351:dbl)
              }
            }
            n195 = flat-sequence {
              tunnel: w342 -> [w350]
              tunnel: [w347] -> w345
              frame #0 {
                # "Repetition 5"
                n196 = call "Math SubVI - Simple (PCR) (DBG OFF) (SBRTN).vi"("Input"=w350) -> ("Output"=w348:dbl)
                n197 = call "Math SubVI - Medium (PCR) (DBG OFF) (SBRTN).vi"("Input"=w348) -> ("Output"=w349:dbl)
                n198 = call "Math SubVI - Complex (PCR) (DBG OFF) (SBRTN).vi"("Input"=w349) -> ("Output"=w347:dbl)
              }
            }
          }
          frame Enabled {
            # "Case 2: Inline VIs"
            n199 = flat-sequence {
              tunnel: w372 -> [w392]
              tunnel: [w389] -> w371
              frame #0 {
                # "Repetition 1"
                n200 = call "Math SubVI - Simple (PCR) (DBG OFF) (INLN).vi"("Input"=w392) -> ("Output"=w390:dbl)
                n201 = call "Math SubVI - Medium (PCR) (DBG OFF) (INLN).vi"("Input"=w390) -> ("Output"=w391:dbl)
                n202 = call "Math SubVI - Complex (PCR) (DBG OFF) (INLN).vi"("Input"=w391) -> ("Output"=w389:dbl)
              }
            }
            n203 = flat-sequence {
              tunnel: w371 -> [w388]
              tunnel: [w385] -> w370
              frame #0 {
                # "Repetition 2"
                n204 = call "Math SubVI - Simple (PCR) (DBG OFF) (INLN).vi"("Input"=w388) -> ("Output"=w386:dbl)
                n205 = call "Math SubVI - Medium (PCR) (DBG OFF) (INLN).vi"("Input"=w386) -> ("Output"=w387:dbl)
                n206 = call "Math SubVI - Complex (PCR) (DBG OFF) (INLN).vi"("Input"=w387) -> ("Output"=w385:dbl)
              }
            }
            n207 = flat-sequence {
              tunnel: w370 -> [w384]
              tunnel: [w381] -> w369
              frame #0 {
                # "Repetition 3"
                n208 = call "Math SubVI - Simple (PCR) (DBG OFF) (INLN).vi"("Input"=w384) -> ("Output"=w382:dbl)
                n209 = call "Math SubVI - Medium (PCR) (DBG OFF) (INLN).vi"("Input"=w382) -> ("Output"=w383:dbl)
                n210 = call "Math SubVI - Complex (PCR) (DBG OFF) (INLN).vi"("Input"=w383) -> ("Output"=w381:dbl)
              }
            }
            n211 = flat-sequence {
              tunnel: w369 -> [w380]
              tunnel: [w377] -> w368
              frame #0 {
                # "Repetition 4"
                n212 = call "Math SubVI - Simple (PCR) (DBG OFF) (INLN).vi"("Input"=w380) -> ("Output"=w378:dbl)
                n213 = call "Math SubVI - Medium (PCR) (DBG OFF) (INLN).vi"("Input"=w378) -> ("Output"=w379:dbl)
                n214 = call "Math SubVI - Complex (PCR) (DBG OFF) (INLN).vi"("Input"=w379) -> ("Output"=w377:dbl)
              }
            }
            n215 = flat-sequence {
              tunnel: w368 -> [w376]
              tunnel: [w373] -> w367
              frame #0 {
                # "Repetition 5"
                n216 = call "Math SubVI - Simple (PCR) (DBG OFF) (INLN).vi"("Input"=w376) -> ("Output"=w374:dbl)
                n217 = call "Math SubVI - Medium (PCR) (DBG OFF) (INLN).vi"("Input"=w374) -> ("Output"=w375:dbl)
                n218 = call "Math SubVI - Complex (PCR) (DBG OFF) (INLN).vi"("Input"=w375) -> ("Output"=w373:dbl)
              }
            }
          }
        }
        n219 = local read "Stop VI?"() -> (w339:bool)
      }
      n220 = for "Loop 6" {
        tunnel: w48 -> [w284] mode=indexing
        tunnel: [w281] -> w38 mode=indexing
        tunnel: [w282] -> w37
        i -> [w282]
        stop <- w283 stop-if-true
        n221 = disable-structure shown="Enabled" {
          disable-tunnel: w284 -> [w290 w316]
          disable-tunnel: [w289 w311] -> w281
          frame Disabled {
            # "Case 1: Subroutines"
            n222 = flat-sequence {
              tunnel: w290 -> [w310]
              tunnel: [w307] -> w285
              frame #0 {
                # "Repetition 1"
                n223 = call "Math SubVI - Simple (PCR) (DBG OFF) (SBRTN).vi"("Input"=w310) -> ("Output"=w308:dbl)
                n224 = call "Math SubVI - Medium (PCR) (DBG OFF) (SBRTN).vi"("Input"=w308) -> ("Output"=w309:dbl)
                n225 = call "Math SubVI - Complex (PCR) (DBG OFF) (SBRTN).vi"("Input"=w309) -> ("Output"=w307:dbl)
              }
            }
            n226 = flat-sequence {
              tunnel: w285 -> [w306]
              tunnel: [w303] -> w288
              frame #0 {
                # "Repetition 2"
                n227 = call "Math SubVI - Simple (PCR) (DBG OFF) (SBRTN).vi"("Input"=w306) -> ("Output"=w304:dbl)
                n228 = call "Math SubVI - Medium (PCR) (DBG OFF) (SBRTN).vi"("Input"=w304) -> ("Output"=w305:dbl)
                n229 = call "Math SubVI - Complex (PCR) (DBG OFF) (SBRTN).vi"("Input"=w305) -> ("Output"=w303:dbl)
              }
            }
            n230 = flat-sequence {
              tunnel: w288 -> [w302]
              tunnel: [w299] -> w287
              frame #0 {
                # "Repetition 3"
                n231 = call "Math SubVI - Simple (PCR) (DBG OFF) (SBRTN).vi"("Input"=w302) -> ("Output"=w300:dbl)
                n232 = call "Math SubVI - Medium (PCR) (DBG OFF) (SBRTN).vi"("Input"=w300) -> ("Output"=w301:dbl)
                n233 = call "Math SubVI - Complex (PCR) (DBG OFF) (SBRTN).vi"("Input"=w301) -> ("Output"=w299:dbl)
              }
            }
            n234 = flat-sequence {
              tunnel: w287 -> [w298]
              tunnel: [w295] -> w286
              frame #0 {
                # "Repetition 4"
                n235 = call "Math SubVI - Simple (PCR) (DBG OFF) (SBRTN).vi"("Input"=w298) -> ("Output"=w296:dbl)
                n236 = call "Math SubVI - Medium (PCR) (DBG OFF) (SBRTN).vi"("Input"=w296) -> ("Output"=w297:dbl)
                n237 = call "Math SubVI - Complex (PCR) (DBG OFF) (SBRTN).vi"("Input"=w297) -> ("Output"=w295:dbl)
              }
            }
            n238 = flat-sequence {
              tunnel: w286 -> [w294]
              tunnel: [w291] -> w289
              frame #0 {
                # "Repetition 5"
                n239 = call "Math SubVI - Simple (PCR) (DBG OFF) (SBRTN).vi"("Input"=w294) -> ("Output"=w292:dbl)
                n240 = call "Math SubVI - Medium (PCR) (DBG OFF) (SBRTN).vi"("Input"=w292) -> ("Output"=w293:dbl)
                n241 = call "Math SubVI - Complex (PCR) (DBG OFF) (SBRTN).vi"("Input"=w293) -> ("Output"=w291:dbl)
              }
            }
          }
          frame Enabled {
            # "Case 2: Inline VIs"
            n242 = flat-sequence {
              tunnel: w316 -> [w336]
              tunnel: [w333] -> w315
              frame #0 {
                # "Repetition 1"
                n243 = call "Math SubVI - Simple (PCR) (DBG OFF) (INLN).vi"("Input"=w336) -> ("Output"=w334:dbl)
                n244 = call "Math SubVI - Medium (PCR) (DBG OFF) (INLN).vi"("Input"=w334) -> ("Output"=w335:dbl)
                n245 = call "Math SubVI - Complex (PCR) (DBG OFF) (INLN).vi"("Input"=w335) -> ("Output"=w333:dbl)
              }
            }
            n246 = flat-sequence {
              tunnel: w315 -> [w332]
              tunnel: [w329] -> w314
              frame #0 {
                # "Repetition 2"
                n247 = call "Math SubVI - Simple (PCR) (DBG OFF) (INLN).vi"("Input"=w332) -> ("Output"=w330:dbl)
                n248 = call "Math SubVI - Medium (PCR) (DBG OFF) (INLN).vi"("Input"=w330) -> ("Output"=w331:dbl)
                n249 = call "Math SubVI - Complex (PCR) (DBG OFF) (INLN).vi"("Input"=w331) -> ("Output"=w329:dbl)
              }
            }
            n250 = flat-sequence {
              tunnel: w314 -> [w328]
              tunnel: [w325] -> w313
              frame #0 {
                # "Repetition 3"
                n251 = call "Math SubVI - Simple (PCR) (DBG OFF) (INLN).vi"("Input"=w328) -> ("Output"=w326:dbl)
                n252 = call "Math SubVI - Medium (PCR) (DBG OFF) (INLN).vi"("Input"=w326) -> ("Output"=w327:dbl)
                n253 = call "Math SubVI - Complex (PCR) (DBG OFF) (INLN).vi"("Input"=w327) -> ("Output"=w325:dbl)
              }
            }
            n254 = flat-sequence {
              tunnel: w313 -> [w324]
              tunnel: [w321] -> w312
              frame #0 {
                # "Repetition 4"
                n255 = call "Math SubVI - Simple (PCR) (DBG OFF) (INLN).vi"("Input"=w324) -> ("Output"=w322:dbl)
                n256 = call "Math SubVI - Medium (PCR) (DBG OFF) (INLN).vi"("Input"=w322) -> ("Output"=w323:dbl)
                n257 = call "Math SubVI - Complex (PCR) (DBG OFF) (INLN).vi"("Input"=w323) -> ("Output"=w321:dbl)
              }
            }
            n258 = flat-sequence {
              tunnel: w312 -> [w320]
              tunnel: [w317] -> w311
              frame #0 {
                # "Repetition 5"
                n259 = call "Math SubVI - Simple (PCR) (DBG OFF) (INLN).vi"("Input"=w320) -> ("Output"=w318:dbl)
                n260 = call "Math SubVI - Medium (PCR) (DBG OFF) (INLN).vi"("Input"=w318) -> ("Output"=w319:dbl)
                n261 = call "Math SubVI - Complex (PCR) (DBG OFF) (INLN).vi"("Input"=w319) -> ("Output"=w317:dbl)
              }
            }
          }
        }
        n262 = local read "Stop VI?"() -> (w283:bool)
      }
      n263 = for "Loop 7" {
        tunnel: w48 -> [w228] mode=indexing
        tunnel: [w225] -> w36 mode=indexing
        tunnel: [w226] -> w35
        i -> [w226]
        stop <- w227 stop-if-true
        n264 = disable-structure shown="Enabled" {
          disable-tunnel: w228 -> [w234 w260]
          disable-tunnel: [w233 w255] -> w225
          frame Disabled {
            # "Case 1: Subroutines"
            n265 = flat-sequence {
              tunnel: w234 -> [w254]
              tunnel: [w251] -> w229
              frame #0 {
                # "Repetition 1"
                n266 = call "Math SubVI - Simple (PCR) (DBG OFF) (SBRTN).vi"("Input"=w254) -> ("Output"=w252:dbl)
                n267 = call "Math SubVI - Medium (PCR) (DBG OFF) (SBRTN).vi"("Input"=w252) -> ("Output"=w253:dbl)
                n268 = call "Math SubVI - Complex (PCR) (DBG OFF) (SBRTN).vi"("Input"=w253) -> ("Output"=w251:dbl)
              }
            }
            n269 = flat-sequence {
              tunnel: w229 -> [w250]
              tunnel: [w247] -> w232
              frame #0 {
                # "Repetition 2"
                n270 = call "Math SubVI - Simple (PCR) (DBG OFF) (SBRTN).vi"("Input"=w250) -> ("Output"=w248:dbl)
                n271 = call "Math SubVI - Medium (PCR) (DBG OFF) (SBRTN).vi"("Input"=w248) -> ("Output"=w249:dbl)
                n272 = call "Math SubVI - Complex (PCR) (DBG OFF) (SBRTN).vi"("Input"=w249) -> ("Output"=w247:dbl)
              }
            }
            n273 = flat-sequence {
              tunnel: w232 -> [w246]
              tunnel: [w243] -> w231
              frame #0 {
                # "Repetition 3"
                n274 = call "Math SubVI - Simple (PCR) (DBG OFF) (SBRTN).vi"("Input"=w246) -> ("Output"=w244:dbl)
                n275 = call "Math SubVI - Medium (PCR) (DBG OFF) (SBRTN).vi"("Input"=w244) -> ("Output"=w245:dbl)
                n276 = call "Math SubVI - Complex (PCR) (DBG OFF) (SBRTN).vi"("Input"=w245) -> ("Output"=w243:dbl)
              }
            }
            n277 = flat-sequence {
              tunnel: w231 -> [w242]
              tunnel: [w239] -> w230
              frame #0 {
                # "Repetition 4"
                n278 = call "Math SubVI - Simple (PCR) (DBG OFF) (SBRTN).vi"("Input"=w242) -> ("Output"=w240:dbl)
                n279 = call "Math SubVI - Medium (PCR) (DBG OFF) (SBRTN).vi"("Input"=w240) -> ("Output"=w241:dbl)
                n280 = call "Math SubVI - Complex (PCR) (DBG OFF) (SBRTN).vi"("Input"=w241) -> ("Output"=w239:dbl)
              }
            }
            n281 = flat-sequence {
              tunnel: w230 -> [w238]
              tunnel: [w235] -> w233
              frame #0 {
                # "Repetition 5"
                n282 = call "Math SubVI - Simple (PCR) (DBG OFF) (SBRTN).vi"("Input"=w238) -> ("Output"=w236:dbl)
                n283 = call "Math SubVI - Medium (PCR) (DBG OFF) (SBRTN).vi"("Input"=w236) -> ("Output"=w237:dbl)
                n284 = call "Math SubVI - Complex (PCR) (DBG OFF) (SBRTN).vi"("Input"=w237) -> ("Output"=w235:dbl)
              }
            }
          }
          frame Enabled {
            # "Case 2: Inline VIs"
            n285 = flat-sequence {
              tunnel: w260 -> [w280]
              tunnel: [w277] -> w259
              frame #0 {
                # "Repetition 1"
                n286 = call "Math SubVI - Simple (PCR) (DBG OFF) (INLN).vi"("Input"=w280) -> ("Output"=w278:dbl)
                n287 = call "Math SubVI - Medium (PCR) (DBG OFF) (INLN).vi"("Input"=w278) -> ("Output"=w279:dbl)
                n288 = call "Math SubVI - Complex (PCR) (DBG OFF) (INLN).vi"("Input"=w279) -> ("Output"=w277:dbl)
              }
            }
            n289 = flat-sequence {
              tunnel: w259 -> [w276]
              tunnel: [w273] -> w258
              frame #0 {
                # "Repetition 2"
                n290 = call "Math SubVI - Simple (PCR) (DBG OFF) (INLN).vi"("Input"=w276) -> ("Output"=w274:dbl)
                n291 = call "Math SubVI - Medium (PCR) (DBG OFF) (INLN).vi"("Input"=w274) -> ("Output"=w275:dbl)
                n292 = call "Math SubVI - Complex (PCR) (DBG OFF) (INLN).vi"("Input"=w275) -> ("Output"=w273:dbl)
              }
            }
            n293 = flat-sequence {
              tunnel: w258 -> [w272]
              tunnel: [w269] -> w257
              frame #0 {
                # "Repetition 3"
                n294 = call "Math SubVI - Simple (PCR) (DBG OFF) (INLN).vi"("Input"=w272) -> ("Output"=w270:dbl)
                n295 = call "Math SubVI - Medium (PCR) (DBG OFF) (INLN).vi"("Input"=w270) -> ("Output"=w271:dbl)
                n296 = call "Math SubVI - Complex (PCR) (DBG OFF) (INLN).vi"("Input"=w271) -> ("Output"=w269:dbl)
              }
            }
            n297 = flat-sequence {
              tunnel: w257 -> [w268]
              tunnel: [w265] -> w256
              frame #0 {
                # "Repetition 4"
                n298 = call "Math SubVI - Simple (PCR) (DBG OFF) (INLN).vi"("Input"=w268) -> ("Output"=w266:dbl)
                n299 = call "Math SubVI - Medium (PCR) (DBG OFF) (INLN).vi"("Input"=w266) -> ("Output"=w267:dbl)
                n300 = call "Math SubVI - Complex (PCR) (DBG OFF) (INLN).vi"("Input"=w267) -> ("Output"=w265:dbl)
              }
            }
            n301 = flat-sequence {
              tunnel: w256 -> [w264]
              tunnel: [w261] -> w255
              frame #0 {
                # "Repetition 5"
                n302 = call "Math SubVI - Simple (PCR) (DBG OFF) (INLN).vi"("Input"=w264) -> ("Output"=w262:dbl)
                n303 = call "Math SubVI - Medium (PCR) (DBG OFF) (INLN).vi"("Input"=w262) -> ("Output"=w263:dbl)
                n304 = call "Math SubVI - Complex (PCR) (DBG OFF) (INLN).vi"("Input"=w263) -> ("Output"=w261:dbl)
              }
            }
          }
        }
        n305 = local read "Stop VI?"() -> (w227:bool)
      }
      n306 = for "Loop 8" {
        tunnel: w48 -> [w172] mode=indexing
        tunnel: [w169] -> w34 mode=indexing
        tunnel: [w170] -> w33
        i -> [w170]
        stop <- w171 stop-if-true
        n307 = disable-structure shown="Enabled" {
          disable-tunnel: w172 -> [w178 w204]
          disable-tunnel: [w177 w199] -> w169
          frame Disabled {
            # "Case 1: Subroutines"
            n308 = flat-sequence {
              tunnel: w178 -> [w198]
              tunnel: [w195] -> w173
              frame #0 {
                # "Repetition 1"
                n309 = call "Math SubVI - Simple (PCR) (DBG OFF) (SBRTN).vi"("Input"=w198) -> ("Output"=w196:dbl)
                n310 = call "Math SubVI - Medium (PCR) (DBG OFF) (SBRTN).vi"("Input"=w196) -> ("Output"=w197:dbl)
                n311 = call "Math SubVI - Complex (PCR) (DBG OFF) (SBRTN).vi"("Input"=w197) -> ("Output"=w195:dbl)
              }
            }
            n312 = flat-sequence {
              tunnel: w173 -> [w194]
              tunnel: [w191] -> w176
              frame #0 {
                # "Repetition 2"
                n313 = call "Math SubVI - Simple (PCR) (DBG OFF) (SBRTN).vi"("Input"=w194) -> ("Output"=w192:dbl)
                n314 = call "Math SubVI - Medium (PCR) (DBG OFF) (SBRTN).vi"("Input"=w192) -> ("Output"=w193:dbl)
                n315 = call "Math SubVI - Complex (PCR) (DBG OFF) (SBRTN).vi"("Input"=w193) -> ("Output"=w191:dbl)
              }
            }
            n316 = flat-sequence {
              tunnel: w176 -> [w190]
              tunnel: [w187] -> w175
              frame #0 {
                # "Repetition 3"
                n317 = call "Math SubVI - Simple (PCR) (DBG OFF) (SBRTN).vi"("Input"=w190) -> ("Output"=w188:dbl)
                n318 = call "Math SubVI - Medium (PCR) (DBG OFF) (SBRTN).vi"("Input"=w188) -> ("Output"=w189:dbl)
                n319 = call "Math SubVI - Complex (PCR) (DBG OFF) (SBRTN).vi"("Input"=w189) -> ("Output"=w187:dbl)
              }
            }
            n320 = flat-sequence {
              tunnel: w175 -> [w186]
              tunnel: [w183] -> w174
              frame #0 {
                # "Repetition 4"
                n321 = call "Math SubVI - Simple (PCR) (DBG OFF) (SBRTN).vi"("Input"=w186) -> ("Output"=w184:dbl)
                n322 = call "Math SubVI - Medium (PCR) (DBG OFF) (SBRTN).vi"("Input"=w184) -> ("Output"=w185:dbl)
                n323 = call "Math SubVI - Complex (PCR) (DBG OFF) (SBRTN).vi"("Input"=w185) -> ("Output"=w183:dbl)
              }
            }
            n324 = flat-sequence {
              tunnel: w174 -> [w182]
              tunnel: [w179] -> w177
              frame #0 {
                # "Repetition 5"
                n325 = call "Math SubVI - Simple (PCR) (DBG OFF) (SBRTN).vi"("Input"=w182) -> ("Output"=w180:dbl)
                n326 = call "Math SubVI - Medium (PCR) (DBG OFF) (SBRTN).vi"("Input"=w180) -> ("Output"=w181:dbl)
                n327 = call "Math SubVI - Complex (PCR) (DBG OFF) (SBRTN).vi"("Input"=w181) -> ("Output"=w179:dbl)
              }
            }
          }
          frame Enabled {
            # "Case 2: Inline VIs"
            n328 = flat-sequence {
              tunnel: w204 -> [w224]
              tunnel: [w221] -> w203
              frame #0 {
                # "Repetition 1"
                n329 = call "Math SubVI - Simple (PCR) (DBG OFF) (INLN).vi"("Input"=w224) -> ("Output"=w222:dbl)
                n330 = call "Math SubVI - Medium (PCR) (DBG OFF) (INLN).vi"("Input"=w222) -> ("Output"=w223:dbl)
                n331 = call "Math SubVI - Complex (PCR) (DBG OFF) (INLN).vi"("Input"=w223) -> ("Output"=w221:dbl)
              }
            }
            n332 = flat-sequence {
              tunnel: w203 -> [w220]
              tunnel: [w217] -> w202
              frame #0 {
                # "Repetition 2"
                n333 = call "Math SubVI - Simple (PCR) (DBG OFF) (INLN).vi"("Input"=w220) -> ("Output"=w218:dbl)
                n334 = call "Math SubVI - Medium (PCR) (DBG OFF) (INLN).vi"("Input"=w218) -> ("Output"=w219:dbl)
                n335 = call "Math SubVI - Complex (PCR) (DBG OFF) (INLN).vi"("Input"=w219) -> ("Output"=w217:dbl)
              }
            }
            n336 = flat-sequence {
              tunnel: w202 -> [w216]
              tunnel: [w213] -> w201
              frame #0 {
                # "Repetition 3"
                n337 = call "Math SubVI - Simple (PCR) (DBG OFF) (INLN).vi"("Input"=w216) -> ("Output"=w214:dbl)
                n338 = call "Math SubVI - Medium (PCR) (DBG OFF) (INLN).vi"("Input"=w214) -> ("Output"=w215:dbl)
                n339 = call "Math SubVI - Complex (PCR) (DBG OFF) (INLN).vi"("Input"=w215) -> ("Output"=w213:dbl)
              }
            }
            n340 = flat-sequence {
              tunnel: w201 -> [w212]
              tunnel: [w209] -> w200
              frame #0 {
                # "Repetition 4"
                n341 = call "Math SubVI - Simple (PCR) (DBG OFF) (INLN).vi"("Input"=w212) -> ("Output"=w210:dbl)
                n342 = call "Math SubVI - Medium (PCR) (DBG OFF) (INLN).vi"("Input"=w210) -> ("Output"=w211:dbl)
                n343 = call "Math SubVI - Complex (PCR) (DBG OFF) (INLN).vi"("Input"=w211) -> ("Output"=w209:dbl)
              }
            }
            n344 = flat-sequence {
              tunnel: w200 -> [w208]
              tunnel: [w205] -> w199
              frame #0 {
                # "Repetition 5"
                n345 = call "Math SubVI - Simple (PCR) (DBG OFF) (INLN).vi"("Input"=w208) -> ("Output"=w206:dbl)
                n346 = call "Math SubVI - Medium (PCR) (DBG OFF) (INLN).vi"("Input"=w206) -> ("Output"=w207:dbl)
                n347 = call "Math SubVI - Complex (PCR) (DBG OFF) (INLN).vi"("Input"=w207) -> ("Output"=w205:dbl)
              }
            }
          }
        }
        n348 = local read "Stop VI?"() -> (w171:bool)
      }
      n349 = for "Loop 9" {
        tunnel: w48 -> [w116] mode=indexing
        tunnel: [w113] -> w32 mode=indexing
        tunnel: [w114] -> w31
        i -> [w114]
        stop <- w115 stop-if-true
        n350 = disable-structure shown="Enabled" {
          disable-tunnel: w116 -> [w122 w148]
          disable-tunnel: [w121 w143] -> w113
          frame Disabled {
            # "Case 1: Subroutines"
            n351 = flat-sequence {
              tunnel: w122 -> [w142]
              tunnel: [w139] -> w117
              frame #0 {
                # "Repetition 1"
                n352 = call "Math SubVI - Simple (PCR) (DBG OFF) (SBRTN).vi"("Input"=w142) -> ("Output"=w140:dbl)
                n353 = call "Math SubVI - Medium (PCR) (DBG OFF) (SBRTN).vi"("Input"=w140) -> ("Output"=w141:dbl)
                n354 = call "Math SubVI - Complex (PCR) (DBG OFF) (SBRTN).vi"("Input"=w141) -> ("Output"=w139:dbl)
              }
            }
            n355 = flat-sequence {
              tunnel: w117 -> [w138]
              tunnel: [w135] -> w120
              frame #0 {
                # "Repetition 2"
                n356 = call "Math SubVI - Simple (PCR) (DBG OFF) (SBRTN).vi"("Input"=w138) -> ("Output"=w136:dbl)
                n357 = call "Math SubVI - Medium (PCR) (DBG OFF) (SBRTN).vi"("Input"=w136) -> ("Output"=w137:dbl)
                n358 = call "Math SubVI - Complex (PCR) (DBG OFF) (SBRTN).vi"("Input"=w137) -> ("Output"=w135:dbl)
              }
            }
            n359 = flat-sequence {
              tunnel: w120 -> [w134]
              tunnel: [w131] -> w119
              frame #0 {
                # "Repetition 3"
                n360 = call "Math SubVI - Simple (PCR) (DBG OFF) (SBRTN).vi"("Input"=w134) -> ("Output"=w132:dbl)
                n361 = call "Math SubVI - Medium (PCR) (DBG OFF) (SBRTN).vi"("Input"=w132) -> ("Output"=w133:dbl)
                n362 = call "Math SubVI - Complex (PCR) (DBG OFF) (SBRTN).vi"("Input"=w133) -> ("Output"=w131:dbl)
              }
            }
            n363 = flat-sequence {
              tunnel: w119 -> [w130]
              tunnel: [w127] -> w118
              frame #0 {
                # "Repetition 4"
                n364 = call "Math SubVI - Simple (PCR) (DBG OFF) (SBRTN).vi"("Input"=w130) -> ("Output"=w128:dbl)
                n365 = call "Math SubVI - Medium (PCR) (DBG OFF) (SBRTN).vi"("Input"=w128) -> ("Output"=w129:dbl)
                n366 = call "Math SubVI - Complex (PCR) (DBG OFF) (SBRTN).vi"("Input"=w129) -> ("Output"=w127:dbl)
              }
            }
            n367 = flat-sequence {
              tunnel: w118 -> [w126]
              tunnel: [w123] -> w121
              frame #0 {
                # "Repetition 5"
                n368 = call "Math SubVI - Simple (PCR) (DBG OFF) (SBRTN).vi"("Input"=w126) -> ("Output"=w124:dbl)
                n369 = call "Math SubVI - Medium (PCR) (DBG OFF) (SBRTN).vi"("Input"=w124) -> ("Output"=w125:dbl)
                n370 = call "Math SubVI - Complex (PCR) (DBG OFF) (SBRTN).vi"("Input"=w125) -> ("Output"=w123:dbl)
              }
            }
          }
          frame Enabled {
            # "Case 2: Inline VIs"
            n371 = flat-sequence {
              tunnel: w148 -> [w168]
              tunnel: [w165] -> w147
              frame #0 {
                # "Repetition 1"
                n372 = call "Math SubVI - Simple (PCR) (DBG OFF) (INLN).vi"("Input"=w168) -> ("Output"=w166:dbl)
                n373 = call "Math SubVI - Medium (PCR) (DBG OFF) (INLN).vi"("Input"=w166) -> ("Output"=w167:dbl)
                n374 = call "Math SubVI - Complex (PCR) (DBG OFF) (INLN).vi"("Input"=w167) -> ("Output"=w165:dbl)
              }
            }
            n375 = flat-sequence {
              tunnel: w147 -> [w164]
              tunnel: [w161] -> w146
              frame #0 {
                # "Repetition 2"
                n376 = call "Math SubVI - Simple (PCR) (DBG OFF) (INLN).vi"("Input"=w164) -> ("Output"=w162:dbl)
                n377 = call "Math SubVI - Medium (PCR) (DBG OFF) (INLN).vi"("Input"=w162) -> ("Output"=w163:dbl)
                n378 = call "Math SubVI - Complex (PCR) (DBG OFF) (INLN).vi"("Input"=w163) -> ("Output"=w161:dbl)
              }
            }
            n379 = flat-sequence {
              tunnel: w146 -> [w160]
              tunnel: [w157] -> w145
              frame #0 {
                # "Repetition 3"
                n380 = call "Math SubVI - Simple (PCR) (DBG OFF) (INLN).vi"("Input"=w160) -> ("Output"=w158:dbl)
                n381 = call "Math SubVI - Medium (PCR) (DBG OFF) (INLN).vi"("Input"=w158) -> ("Output"=w159:dbl)
                n382 = call "Math SubVI - Complex (PCR) (DBG OFF) (INLN).vi"("Input"=w159) -> ("Output"=w157:dbl)
              }
            }
            n383 = flat-sequence {
              tunnel: w145 -> [w156]
              tunnel: [w153] -> w144
              frame #0 {
                # "Repetition 4"
                n384 = call "Math SubVI - Simple (PCR) (DBG OFF) (INLN).vi"("Input"=w156) -> ("Output"=w154:dbl)
                n385 = call "Math SubVI - Medium (PCR) (DBG OFF) (INLN).vi"("Input"=w154) -> ("Output"=w155:dbl)
                n386 = call "Math SubVI - Complex (PCR) (DBG OFF) (INLN).vi"("Input"=w155) -> ("Output"=w153:dbl)
              }
            }
            n387 = flat-sequence {
              tunnel: w144 -> [w152]
              tunnel: [w149] -> w143
              frame #0 {
                # "Repetition 5"
                n388 = call "Math SubVI - Simple (PCR) (DBG OFF) (INLN).vi"("Input"=w152) -> ("Output"=w150:dbl)
                n389 = call "Math SubVI - Medium (PCR) (DBG OFF) (INLN).vi"("Input"=w150) -> ("Output"=w151:dbl)
                n390 = call "Math SubVI - Complex (PCR) (DBG OFF) (INLN).vi"("Input"=w151) -> ("Output"=w149:dbl)
              }
            }
          }
        }
        n391 = local read "Stop VI?"() -> (w115:bool)
      }
      n392 = for "Loop 10" {
        tunnel: w48 -> [w60] mode=indexing
        tunnel: [w57] -> w30 mode=indexing
        tunnel: [w58] -> w29
        i -> [w58]
        stop <- w59 stop-if-true
        n393 = disable-structure shown="Enabled" {
          disable-tunnel: w60 -> [w66 w92]
          disable-tunnel: [w65 w87] -> w57
          frame Disabled {
            # "Case 1: Subroutines"
            n394 = flat-sequence {
              tunnel: w66 -> [w86]
              tunnel: [w83] -> w61
              frame #0 {
                # "Repetition 1"
                n395 = call "Math SubVI - Simple (PCR) (DBG OFF) (SBRTN).vi"("Input"=w86) -> ("Output"=w84:dbl)
                n396 = call "Math SubVI - Medium (PCR) (DBG OFF) (SBRTN).vi"("Input"=w84) -> ("Output"=w85:dbl)
                n397 = call "Math SubVI - Complex (PCR) (DBG OFF) (SBRTN).vi"("Input"=w85) -> ("Output"=w83:dbl)
              }
            }
            n398 = flat-sequence {
              tunnel: w61 -> [w82]
              tunnel: [w79] -> w64
              frame #0 {
                # "Repetition 2"
                n399 = call "Math SubVI - Simple (PCR) (DBG OFF) (SBRTN).vi"("Input"=w82) -> ("Output"=w80:dbl)
                n400 = call "Math SubVI - Medium (PCR) (DBG OFF) (SBRTN).vi"("Input"=w80) -> ("Output"=w81:dbl)
                n401 = call "Math SubVI - Complex (PCR) (DBG OFF) (SBRTN).vi"("Input"=w81) -> ("Output"=w79:dbl)
              }
            }
            n402 = flat-sequence {
              tunnel: w64 -> [w78]
              tunnel: [w75] -> w63
              frame #0 {
                # "Repetition 3"
                n403 = call "Math SubVI - Simple (PCR) (DBG OFF) (SBRTN).vi"("Input"=w78) -> ("Output"=w76:dbl)
                n404 = call "Math SubVI - Medium (PCR) (DBG OFF) (SBRTN).vi"("Input"=w76) -> ("Output"=w77:dbl)
                n405 = call "Math SubVI - Complex (PCR) (DBG OFF) (SBRTN).vi"("Input"=w77) -> ("Output"=w75:dbl)
              }
            }
            n406 = flat-sequence {
              tunnel: w63 -> [w74]
              tunnel: [w71] -> w62
              frame #0 {
                # "Repetition 4"
                n407 = call "Math SubVI - Simple (PCR) (DBG OFF) (SBRTN).vi"("Input"=w74) -> ("Output"=w72:dbl)
                n408 = call "Math SubVI - Medium (PCR) (DBG OFF) (SBRTN).vi"("Input"=w72) -> ("Output"=w73:dbl)
                n409 = call "Math SubVI - Complex (PCR) (DBG OFF) (SBRTN).vi"("Input"=w73) -> ("Output"=w71:dbl)
              }
            }
            n410 = flat-sequence {
              tunnel: w62 -> [w70]
              tunnel: [w67] -> w65
              frame #0 {
                # "Repetition 5"
                n411 = call "Math SubVI - Simple (PCR) (DBG OFF) (SBRTN).vi"("Input"=w70) -> ("Output"=w68:dbl)
                n412 = call "Math SubVI - Medium (PCR) (DBG OFF) (SBRTN).vi"("Input"=w68) -> ("Output"=w69:dbl)
                n413 = call "Math SubVI - Complex (PCR) (DBG OFF) (SBRTN).vi"("Input"=w69) -> ("Output"=w67:dbl)
              }
            }
          }
          frame Enabled {
            # "Case 2: Inline VIs"
            n414 = flat-sequence {
              tunnel: w92 -> [w112]
              tunnel: [w109] -> w91
              frame #0 {
                # "Repetition 1"
                n415 = call "Math SubVI - Simple (PCR) (DBG OFF) (INLN).vi"("Input"=w112) -> ("Output"=w110:dbl)
                n416 = call "Math SubVI - Medium (PCR) (DBG OFF) (INLN).vi"("Input"=w110) -> ("Output"=w111:dbl)
                n417 = call "Math SubVI - Complex (PCR) (DBG OFF) (INLN).vi"("Input"=w111) -> ("Output"=w109:dbl)
              }
            }
            n418 = flat-sequence {
              tunnel: w91 -> [w108]
              tunnel: [w105] -> w90
              frame #0 {
                # "Repetition 2"
                n419 = call "Math SubVI - Simple (PCR) (DBG OFF) (INLN).vi"("Input"=w108) -> ("Output"=w106:dbl)
                n420 = call "Math SubVI - Medium (PCR) (DBG OFF) (INLN).vi"("Input"=w106) -> ("Output"=w107:dbl)
                n421 = call "Math SubVI - Complex (PCR) (DBG OFF) (INLN).vi"("Input"=w107) -> ("Output"=w105:dbl)
              }
            }
            n422 = flat-sequence {
              tunnel: w90 -> [w104]
              tunnel: [w101] -> w89
              frame #0 {
                # "Repetition 3"
                n423 = call "Math SubVI - Simple (PCR) (DBG OFF) (INLN).vi"("Input"=w104) -> ("Output"=w102:dbl)
                n424 = call "Math SubVI - Medium (PCR) (DBG OFF) (INLN).vi"("Input"=w102) -> ("Output"=w103:dbl)
                n425 = call "Math SubVI - Complex (PCR) (DBG OFF) (INLN).vi"("Input"=w103) -> ("Output"=w101:dbl)
              }
            }
            n426 = flat-sequence {
              tunnel: w89 -> [w100]
              tunnel: [w97] -> w88
              frame #0 {
                # "Repetition 4"
                n427 = call "Math SubVI - Simple (PCR) (DBG OFF) (INLN).vi"("Input"=w100) -> ("Output"=w98:dbl)
                n428 = call "Math SubVI - Medium (PCR) (DBG OFF) (INLN).vi"("Input"=w98) -> ("Output"=w99:dbl)
                n429 = call "Math SubVI - Complex (PCR) (DBG OFF) (INLN).vi"("Input"=w99) -> ("Output"=w97:dbl)
              }
            }
            n430 = flat-sequence {
              tunnel: w88 -> [w96]
              tunnel: [w93] -> w87
              frame #0 {
                # "Repetition 5"
                n431 = call "Math SubVI - Simple (PCR) (DBG OFF) (INLN).vi"("Input"=w96) -> ("Output"=w94:dbl)
                n432 = call "Math SubVI - Medium (PCR) (DBG OFF) (INLN).vi"("Input"=w94) -> ("Output"=w95:dbl)
                n433 = call "Math SubVI - Complex (PCR) (DBG OFF) (INLN).vi"("Input"=w95) -> ("Output"=w93:dbl)
              }
            }
          }
        }
        n434 = local read "Stop VI?"() -> (w59:bool)
      }
      n435 = flat-sequence {
        tunnel: w55 -> [w617]
        frame #0 {
          n436 = call <vilib>:"Clear Errors.vi"("error in (no error)"=w617) -> ()  [unwired: 5 in, 2 out]
          "Stop VI?" <- TRUE
        }
      }
      n437 = Increment(x=w40) -> (x+1=w39:i32)
      n438 = Increment(x=w37) -> (x+1=w24:i32)
      n439 = Increment(x=w35) -> (x+1=w25:i32)
      n440 = Increment(x=w33) -> (x+1=w26:i32)
      n441 = Increment(x=w31) -> (x+1=w27:i32)
      n442 = Increment(x=w29) -> (x+1=w28:i32)
      n443 = Increment(x=w53) -> (x+1=w52:i32)
      n444 = Increment(x=w47) -> (x+1=w51:i32)
      n445 = Increment(x=w45) -> (x+1=w50:i32)
      n446 = Increment(x=w43) -> (x+1=w49:i32)
    }
    frame #2 {
      n447 = Build Array(w640, w639, w634, w633, w624, w623, w622, w621, w620, w619) -> (w632:i32[])
      n448 = To Double Precision Float(number=w632) -> (double precision float=w631:dbl[])
      n449 = call-poly <vilib>:"Mean.vi"("X"=w631) -> ("mean"=w638:dbl)  [unwired: 1 out]
      "Avg. No. Of Iterations Executed - All Loops" <- w638
      n450 = call "Copy Result To Clipboard.vi"("No. Of Decimal Places (6)"=u32 1, "Input"=w638) -> ()
      "No. Of Iterations Executed - Loop 1" <- w640
      "Output - Loop 1" <- w642
      "No. Of Iterations Executed - Loop 2" <- w639
      "Output - Loop 2" <- w641
      "No. Of Iterations Executed - Loop 3" <- w634
      "Output - Loop 3" <- w637
      "No. Of Iterations Executed - Loop 4" <- w633
      "Output - Loop 4" <- w636
      "No. Of Iterations Executed - Loop 5" <- w624
      "Output - Loop 5" <- w630
      "No. Of Iterations Executed - Loop 6" <- w623
      "Output - Loop 6" <- w629
      "No. Of Iterations Executed - Loop 7" <- w622
      "Output - Loop 7" <- w628
      "No. Of Iterations Executed - Loop 8" <- w621
      "Output - Loop 8" <- w627
      "No. Of Iterations Executed - Loop 9" <- w620
      "Output - Loop 9" <- w626
      "No. Of Iterations Executed - Loop 10" <- w619
      "Output - Loop 10" <- w625
    }
  }
